vi "Get FPGA Data - Local.vi"(8 "error in (no error)":errorcluster, 11 "Item Ref in":T1 format="%.0x") -> (0 "error out":errorcluster, 2 "FPGA":T2 {"UDVs"."To FPGA"."VS ref" format="%.0x"; "UDVs"."From FPGA"."VS ref" format="%.0x"; "VS ref" format="%.0x"; "Output Data"."BD Refs"."Data Reference" format="%.0x"; "Input Data"."BD Refs"."Data Reference" format="%.0x"}, 3 "Item Ref out":T1 format="%.0x", 4 "FPGALoaded":bool)   [LabVIEW 2011, in "Scan Engine Custom Device.lvlib"]
uses:
  Scan Engine Custom Device.lvlib
  Type Defs/FPGA Data.ctl
  <vilib>/NI Veristand/Custom Device API/Custom Device Item Ref.ctl
  Type Defs/Input Data.ctl
  <vilib>/NI Veristand/Custom Device API/Block Data Reference.ctl
  <vilib>/NI Veristand/Custom Device API/Data Reference.ctl
  Type Defs/Output Data.ctl
  Type Defs/UDV Data.ctl
  Type Defs/UDV Data Type.ctl
  Type Defs/FXP Config.ctl
  Globals/Property Strings.vi
  <vilib>/NI Veristand/Custom Device API/Get Item Property (String).vi
  <vilib>/NI Veristand/Custom Device API/Get Item Property (Path).vi
  <vilib>/NI Veristand/Custom Device API/Custom Device API.lvlib
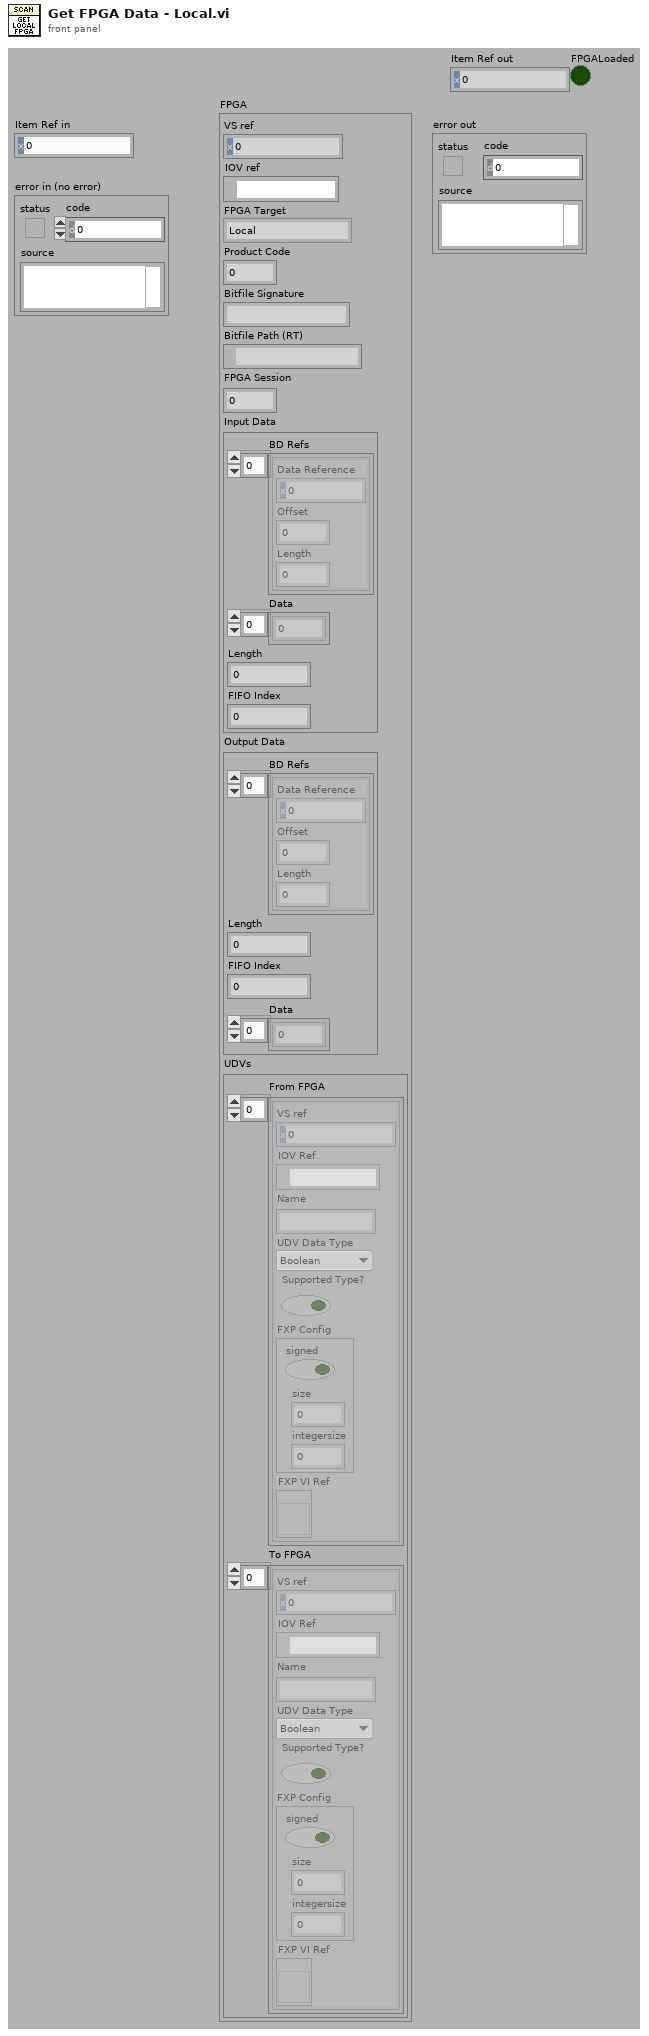
[diagram p1: front panel]
types:
  T1 = typedef "Custom Device API.lvlib/Custom Device Item Ref.ctl" = u64
  T2 = typedef "Scan Engine Custom Device.lvlib/FPGA Data.ctl" = cluster{"VS ref":T1, "IOV ref":refnum<k21>, "FPGA Target":enum16{"Local", "EtherCAT"}, "Product Code":u32, "Bitfile Signature":string, "Bitfile Path (RT)":path, "FPGA Session":u32, "Input Data":T3, "Output Data":T6, "UDVs":cluster{"From FPGA":T7[], "To FPGA":T7[]}}
  T3 = typedef "Scan Engine Custom Device.lvlib/Input Data.ctl" = cluster{"BD Refs":T4[], "Data":dbl[], "Length":i32, "FIFO Index":i32}
  T4 = typedef "Custom Device API.lvlib/Block Data Reference.ctl" = cluster{"Data Reference":T5, "Offset":i32, "Length":i32}
  T5 = typedef "Custom Device API.lvlib/Data Reference.ctl" = i32
  T6 = typedef "Scan Engine Custom Device.lvlib/Output Data.ctl" = cluster{"BD Refs":T4[], "Length":i32, "FIFO Index":i32, "Data":dbl[]}
  T7 = typedef "Scan Engine Custom Device.lvlib/UDV Data.ctl" = cluster{"VS ref":T1, "IOV Ref":refnum<k21>, "Name":string, "UDV Data Type":T8, "Supported Type?":bool, "FXP Config":T9, "FXP VI Ref":refnum<vi>}
  T8 = typedef "Scan Engine Custom Device.lvlib/UDV Data Type.ctl" = enum16{"Boolean", "Fixed Point", "Int8", "Int16", "Int32", "Int64", "U32 Bit Field", "UInt8", "UInt16", "UInt32", "UInt64", "Other"}
  T9 = typedef "Scan Engine Custom Device.lvlib/FXP Config.ctl" = cluster{"signed":bool, "size":u32, "integersize":i32}
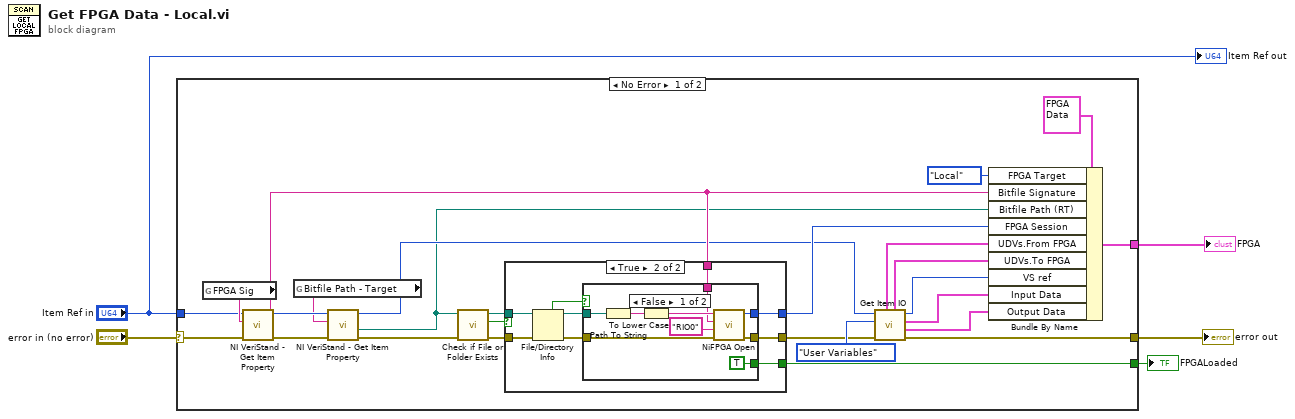
[diagram p0: block diagram]
diagram:
  n1 = case shown="No Error" "error in (no error)" {
    selector: "error in (no error)" -> [w13 w52]
    tunnel: [w31 _] -> w5
    tunnel: [w25 w52] -> w4
    tunnel: "Item Ref in" -> [w14 _]
    tunnel: [w6 _] -> w1
    frame No Error {
      n2 = global read "Property Strings.vi" "FPGA Sig"() -> (w22:string)
      n3 = call-poly <vilib>:"NI VeriStand - Get Item Property.vi"("error in (no error)"=w13, "Property Name"=w22, "Item Ref in"=w14) -> ("error out"=w29:errorcluster, "Value"=w20:string, "Item Ref out"=w30:T1)  [unwired: 5 in, 1 out]
      n4 = global read "Property Strings.vi" "Bitfile Path - Target"() -> (w7:string)
      n5 = call-poly <vilib>:"NI VeriStand - Get Item Property.vi"("error in (no error)"=w29, "Property Name"=w7, "Item Ref in"=w30) -> ("error out"=w9:errorcluster, "Value"=w8:path, "Item Ref out"=w17:T1)  [unwired: 5 in, 1 out]
      n6 = call <vilib>:"Check if File or Folder Exists.vi"("error in (no error)"=w9, "path"=w8) -> ("error out"=w12:errorcluster, "file or folder exists?"=w11:bool, "dup path"=w10:path)  [unwired: 7 in]
      n7 = case shown="True" w11 {
        tunnel: w10 -> [_ w36]
        tunnel: w20 -> [_ w41]
        tunnel: [w32 w40] -> w19
        tunnel: [_ w39] -> w18
        tunnel: w12 -> [w32 w38]
        tunnel: [_ w33] -> w6
        frame False {
        }
        frame True {
          n8 = File/Directory Info(path=w36, error in=w38) -> (path out=w35:path, directory=w34:bool, error out=w37:errorcluster)  [unwired: 4 out]
          n9 = case shown="False" w34 {
            tunnel: w35 -> [w50 _]
            tunnel: w41 -> [w47 _]
            tunnel: [w46 w51] -> w40
            tunnel: [w45 _] -> w39
            tunnel: w37 -> [w44 w51]
            tunnel: [TRUE _] -> w33
            frame False {
              n10 = Path To String(path=w50) -> (string=w43:string)
              n11 = To Lower Case(string=w43) -> (all lower case string=w49:string)
              n12 = call "NiFPGA Open.vi"("error in (no error)"=w44, "Resource"="RIO0", "Signature"=w47, "Bitfile"=w49) -> ("error out"=w46:errorcluster, "Session Out"=w45:u32)  [unwired: 5 in, 1 out]
            }
            frame True {
            }
          }
        }
      }
      n13 = call "Get Item IO.vi"("error in (no error)"=w19, "Item Type"=enum16{"RSI Module", "User Variables"}."User Variables", "Item Ref in"=w17) -> ("error out"=w25:errorcluster, "Output Data"=w23:T6, "Input Data"=w24:T3, "Item Ref out"=w26:T1, "To FPGA"=w15:T7[], "From FPGA"=w16:T7[])  [unwired: 2 in, 1 out]
      n14 = Bundle By Name(cluster=T2 {"VS ref"=0, "IOV ref"="", "FPGA Target"=enum."Local", "Product Code"=0, "Bitfile Signature"="", "Bitfile Path (RT)"=path "", "FPGA Session"=0, "Input Data"={"BD Refs"=[], "Data"=[], "Length"=0, "FIFO Index"=0}, "Output Data"={"BD Refs"=[], "Length"=0, "FIFO Index"=0, "Data"=[]}, "UDVs"={"From FPGA"=[], "To FPGA"=[]}} ("FPGA"), "FPGA Target"=enum16{"Local", "EtherCAT"}."Local", "Bitfile Signature"=w20, "Bitfile Path (RT)"=w8, "FPGA Session"=w18, "UDVs.From FPGA"=w16, "UDVs.To FPGA"=w15, "VS ref"=w26, "Input Data"=w24, "Output Data"=w23) -> (w31:T2)
    }
    frame Error {
    }
  }
  "FPGA" <- w5
  "error out" <- w4
  "FPGALoaded" <- w1
  "Item Ref out" <- "Item Ref in"
